vi "Siemens Wait time.vi"(6 "milliseconds to wait":u32=100, 8 "error in (no error)":errorcluster) -> (0 "error out":errorcluster, 4 "millisecond timer value":u32)   [LabVIEW 2014, in "Simatic S7.lvlib"]
uses:
  Simatic S7.lvlib
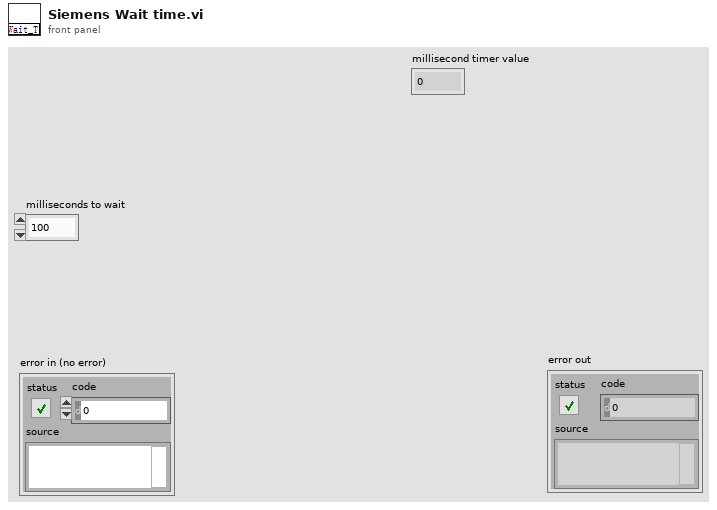
[diagram p1: front panel]
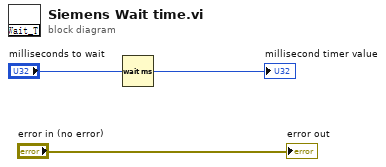
[diagram p0: block diagram]
diagram:
  n1 = Wait (ms)(milliseconds to wait="milliseconds to wait") -> (millisecond timer value=→"millisecond timer value":u32)
  "error out" <- "error in (no error)"
